vi "FetchTargetFile.vi"(6 "file type":T1, 8 "error in (no error)":errorcluster, 10 "FileName":string="MyData", 11 "Target Folder":path) -> (0 "error out":errorcluster, 3 "Full File Path":path)   [LabVIEW 2018, in "RW_Protocols.lvlib"]
uses:
  RW_Protocols.lvlib
  FileType.ctl
panel:
  out "file or folder exists?":bool
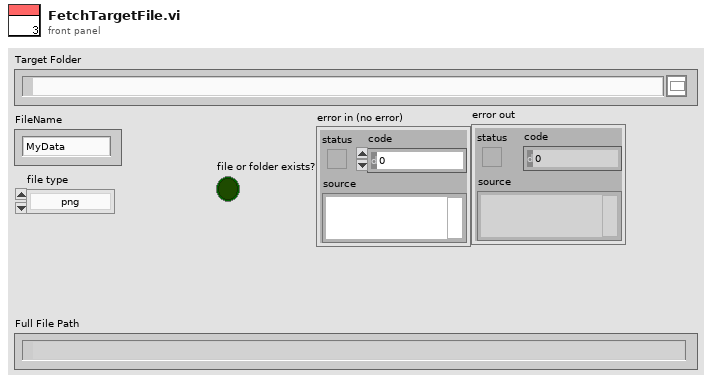
[diagram p1: front panel]
types:
  T1 = typedef "RW_Protocols.lvlib/FileType.ctl" = enum16{"png", "csv", "tiff", "dat", "bin", "txt"}
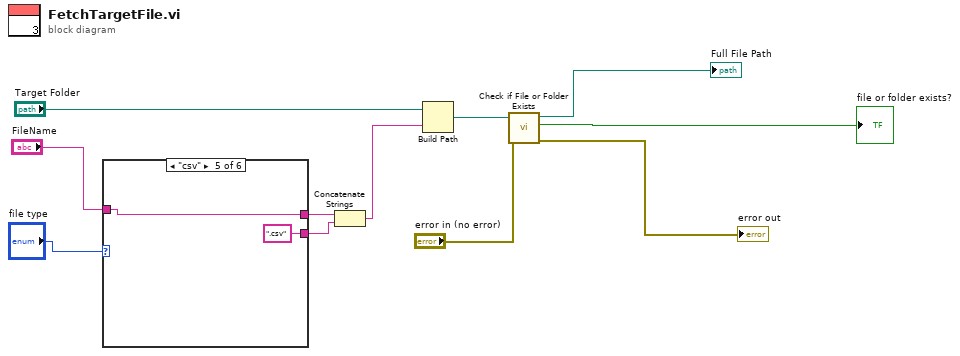
[diagram p0: block diagram]
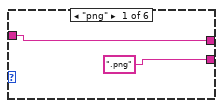
[diagram p2: hidden frame]
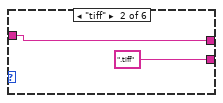
[diagram p3: hidden frame]
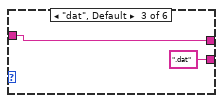
[diagram p4: hidden frame]
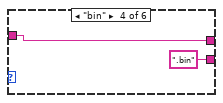
[diagram p5: hidden frame]
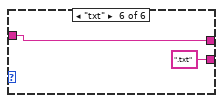
[diagram p6: hidden frame]
diagram:
  n1 = case shown="\"csv\"" "file type" {
    tunnel: "FileName" -> [w13 w15 w17 w19 w21 w23]
    tunnel: [w13 w15 w17 w19 w21 w23] -> w6
    tunnel: [".png" ("string") ".tiff" ("string") ".dat" ("string") ".bin" ("string") ".csv" ("string") ".txt" ("string")] -> w4
    frame "png" {
    }
    frame "tiff" {
    }
    frame "dat", Default {
    }
    frame "bin" {
    }
    frame "csv" {
    }
    frame "txt" {
    }
  }
  n2 = Concatenate Strings(w6, w4) -> (w3:string)
  n3 = Build Path(base path="Target Folder", name or relative path=w3) -> (appended path=w11:path)
  n4 = call <vilib>:"Check if File or Folder Exists.vi"("error in (no error)"="error in (no error)", "path"=w11) -> ("error out"=→"error out":errorcluster, "file or folder exists?"=→"file or folder exists?":bool, "dup path"=→"Full File Path":path)  [unwired: 7 in]
